vi "Destroy.vi"(0 "reference in":refnum<class "G4SubTemplate_Simple_5x6x5.lvclass">, 11 "error in (no error)":errorcluster) -> (4 "reference out":refnum<class "G4SubTemplate_Simple_5x6x5.lvclass">, 15 "error out":errorcluster)   [LabVIEW 2016, in "G4SubTemplate_Simple_5x6x5.lvclass"]
uses:
  <resource>/Framework/Providers/Open_GDS/ClassProviders/Provider_EndevoGOOP400/Templates/G4SubTemplate_Simple_5x6x5/G4SubTemplate_Simple_5x6x5.lvclass
  <resource>/Framework/Providers/Open_GDS/ClassProviders/Provider_EndevoGOOP400/Templates/G4BaseTemplate_Simple_5x6x5/G4BaseTemplate_Simple_5x6x5.lvclass
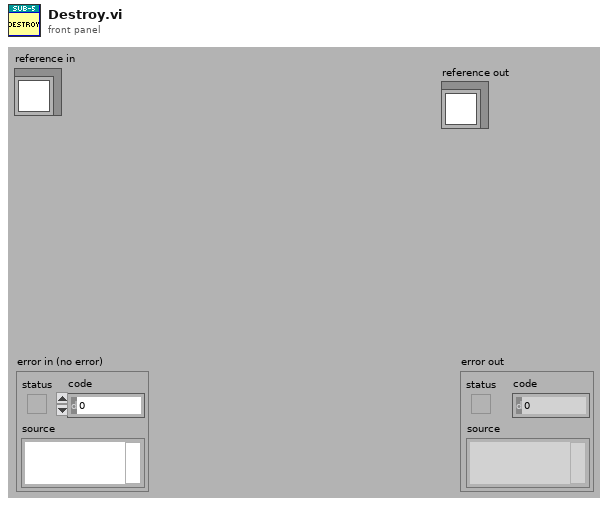
[diagram p1: front panel]
types:
  T1 = typedef "G4SubTemplate_Simple_5x6x5.lvclass/ObjectAttributes.ctl" = cluster{"Attribute1":dbl}
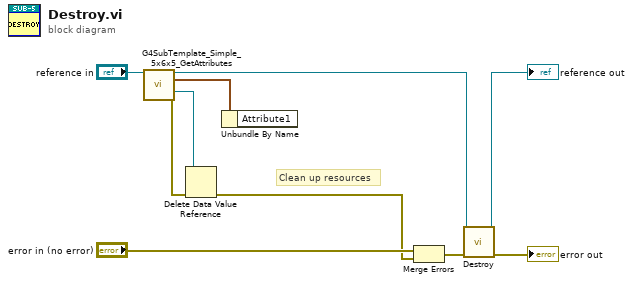
[diagram p0: block diagram]
diagram:
  # "Clean up resources"
  n1 = call <resource>:"G4SubTemplate_Simple_5x6x5_GetAttributes.vi"("reference in"="reference in") -> ("reference out"=w3:refnum<class "G4SubTemplate_Simple_5x6x5.lvclass">, "Data"=w9:T1, "DataRef"=w8:refnum<data-value>, "error out"=w10:errorcluster)  [unwired: 11 in]
  n2 = Delete Data Value Reference(data value reference=w8, error in=w10) -> (error out=w6:errorcluster)  [unwired: 1 out]
  n3 = Unbundle By Name(w9) -> ()  [unwired: 1 out]
  n4 = Merge Errors("error in (no error)", w6) -> (w4:errorcluster)
  n5 = call-parent "Destroy.vi"("reference in"=w3, "error in (no error)"=w4) -> ("reference out"=→"reference out":refnum<class "G4SubTemplate_Simple_5x6x5.lvclass">, "error out"=→"error out":errorcluster)  [unwired: 12 in]
